vi "Set Sensitivity.vi"(9 "Range":u16(ring)=50 items=["10 mm/s"=1, "20 mm/s"=2, "50 mm/s"=5, "100 mm/s"=10, "200 mm/s"=20, "500 mm/s"=50, "1 m/s"=100, "2 m/s"=200], 11 "RS232":refnum<visa-resource-name>="ASRL27::INSTR") -> (0 "Success?":bool, 3 "RS232 out":refnum<visa-resource-name>="ASRL27::INSTR")   [LabVIEW 2022 SP3]
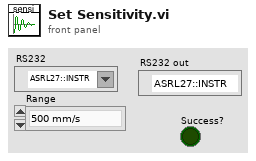
[diagram p1: front panel]
types:
  T1 = enum16{"10 mm/s", "20 mm/s", "50 mm/s", "100 mm/s", "200 mm/s", "500 mm/s", "1 m/s", "2 m/s"}
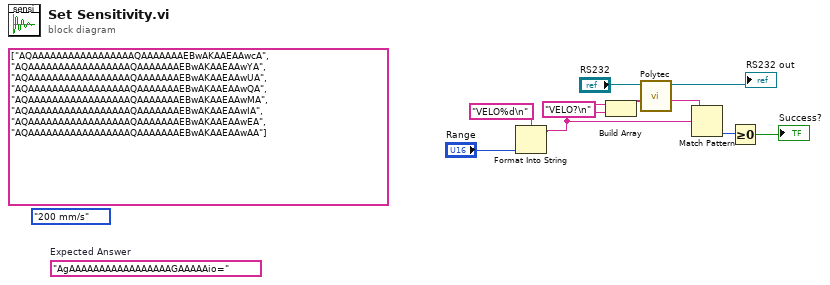
[diagram p0: block diagram]
diagram:
  (unwired) T1."200 mm/s" ("Range")
  (unwired) string[] ["AQAAAAAAAAAAAAAAAAAQAAAAAAAEBwAKAAEAAwcA", "AQAAAAAAAAAAAAAAAAAQAAAAAAAEBwAKAAEAAwYA", "AQAAAAAAAAAAAAAAAAAQAAAAAAAEBwAKAAEAAwUA", "AQAAAAAAAAAAAAAAAAAQAAAAAAAEBwAKAAEAAwQA", "AQAAAAAAAAAAAAAAAAAQAAAAAAAEBwAKAAEAAwMA", "AQAAAAAAAAAAAAAAAAAQAAAAAAAEBwAKAAEAAwIA", "AQAAAAAAAAAAAAAAAAAQAAAAAAAEBwAKAAEAAwEA", "AQAAAAAAAAAAAAAAAAAQAAAAAAAEBwAKAAEAAwAA"]
  (unwired) "AgAAAAAAAAAAAAAAAAAGAAAAAio="  # Expected Answer
  n1 = Format Into String(format string="VELO%d\n", "Range") -> (resulting string=w5:string)  [unwired: 2 in, 1 out]
  n2 = Build Array(w5, "VELO?\n" ("format string")) -> (w2:string[])
  n3 = call "Polytec.vi"("RS232"="RS232", "Strings"=w2) -> ("RS232 out"=→"RS232 out":refnum<visa-resource-name>, "String Read"=w6:string)  [unwired: 7 in]
  n4 = Match Pattern(string=w6, regular expression=w5) -> (offset past match=w4:i32)  [unwired: 1 in, 3 out]
  n5 = Greater Or Equal To 0?(x=w4) -> (x >= 0?=→"Success?":bool)
